vi "Update Values by Index.vi"(4 "Raw":dbl[](array[numeric]), 6 "Timestamp (Now)":dbl, 8 "error in (no error)":errorcluster, 9 "Scaled":dbl[](array[numeric]), 10 "Index":i32[](array[numeric]), 11 "Group in":refnum<class "Group DBL.lvclass">) -> (0 "error out":errorcluster, 3 "Group out":refnum<class "Group DBL.lvclass">)   [LabVIEW 2020, in "Vecto.lvlib" / "Group DBL.lvclass"]
uses:
  Group DBL.lvclass
  C:/dev/lv20CE/relink/lv-vecto/Vecto/Group/Group.lvclass
  Group DBL.lvclass/Group DBL.ctl
  Group/Group.lvclass
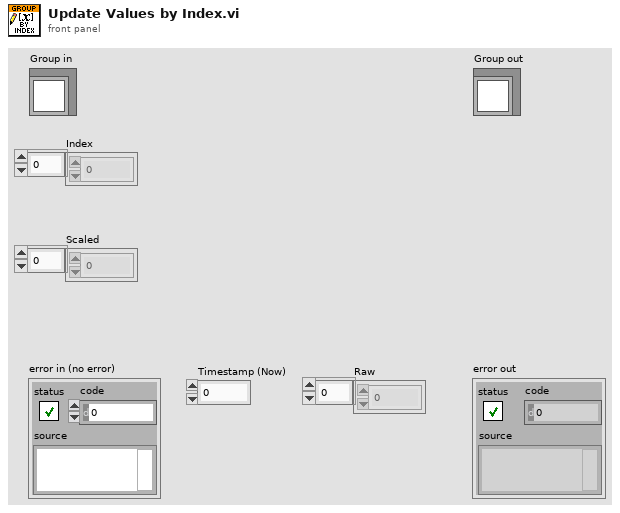
[diagram p1: front panel]
types:
  T1 = typedef "Vecto.lvlib/Group.lvclass/Ref.ctl" = cluster{"Scaled":dbl[], "Timestamp":dbl[], "Raw":dbl[]}
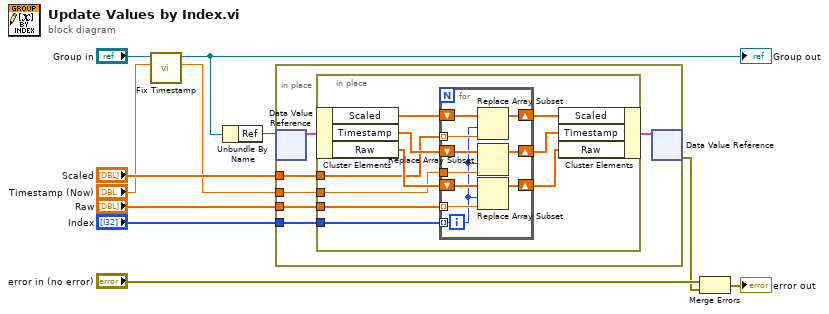
[diagram p0: block diagram]
diagram:
  n1 = call "Fix Timestamp.vi"("Timestamp in"="Timestamp (Now)", "GroupAbstract in"="Group in") -> ("Timestamp"=w1:dbl, "GroupAbstract out"=w3:refnum<class "Group DBL.lvclass">)  [unwired: 7 in, 1 out]
  "Group out" <- w3
  n2 = Unbundle By Name(w3) -> ("Ref"=w10:refnum<data-value>)
  n3 = in-place {
    in-place-border: "Scaled" -> [w16]
    in-place-border: w1 -> [w15]
    in-place-border: "Raw" -> [w14]
    in-place-border: "Index" -> [w13]
    n4 = in-place-dvr #1(w10) -> (w17:T1)  [unwired: 1 out]
    n5 = in-place {
      in-place-border: w16 -> [w22]
      in-place-border: w15 -> [w23]
      in-place-border: w14 -> [w25]
      in-place-border: w13 -> [w18]
      n6 = in-place-cluster #2(w17) -> ("Scaled"=w27:dbl[], "Timestamp"=w24:dbl[], "Raw"=w26:dbl[])
      n7 = for {
        tunnel: w25 -> [w35] mode=indexing
        tunnel: w23 -> [w33]
        tunnel: w22 -> [w32] mode=indexing
        shift-right: [w31] -> w21
        shift-left: w27 -> [w37]
        shift-right: [w30] -> w20
        shift-left: w24 -> [w34]
        shift-right: [w29] -> w19
        shift-left: w26 -> [w36]
        tunnel: w18 -> [w28] mode=indexing
        n8 = Replace Array Subset(array=w37, new element=w32, index=w28) -> (w31:dbl[])
        n9 = Replace Array Subset(array=w34, new element=w33, index=w28) -> (w30:dbl[])
        n10 = Replace Array Subset(array=w36, new element=w35, index=w28) -> (w29:dbl[])
      }
      n11 = in-place-cluster #2("Scaled"=w21, "Timestamp"=w20, "Raw"=w19) -> (w12:T1)
    }
    n12 = in-place-dvr #1(w12) -> (w5:errorcluster)  [unwired: 1 out]
  }
  n13 = Merge Errors("error in (no error)", w5) -> (→"error out":errorcluster)
